vi "Read Background.vi"(8 "error in (no error)":errorcluster, 10 "Path":path, 11 "BigMAQ in":refnum<class "BigMAQ.lvclass">) -> (0 "error out":errorcluster, 3 "BigMAQ out":refnum<class "BigMAQ.lvclass">, 4 "Metadata":variant)   [LabVIEW 2019, in "BigMAQ.lvclass"]
uses:
  BigMAQ.lvclass
  BigMAQ.lvclass/BigMAQ.ctl
  <vilib>/vision/NI_Vision_Development_Module.lvlib
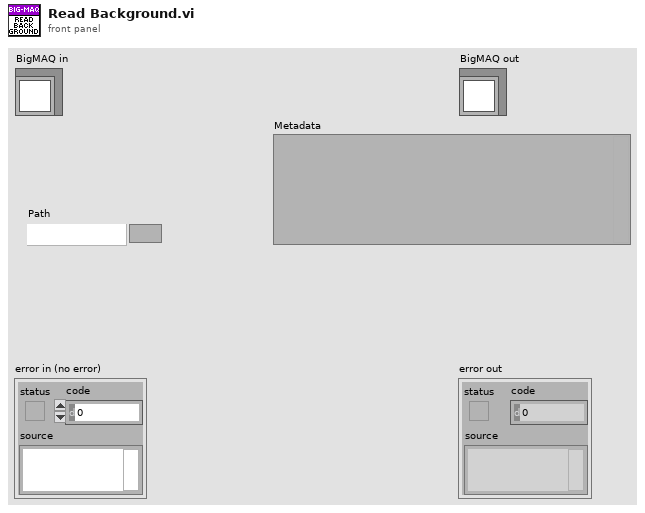
[diagram p1: front panel]
types:
  T1 = typedef "IMAQ Image.ctl" = refnum<image>
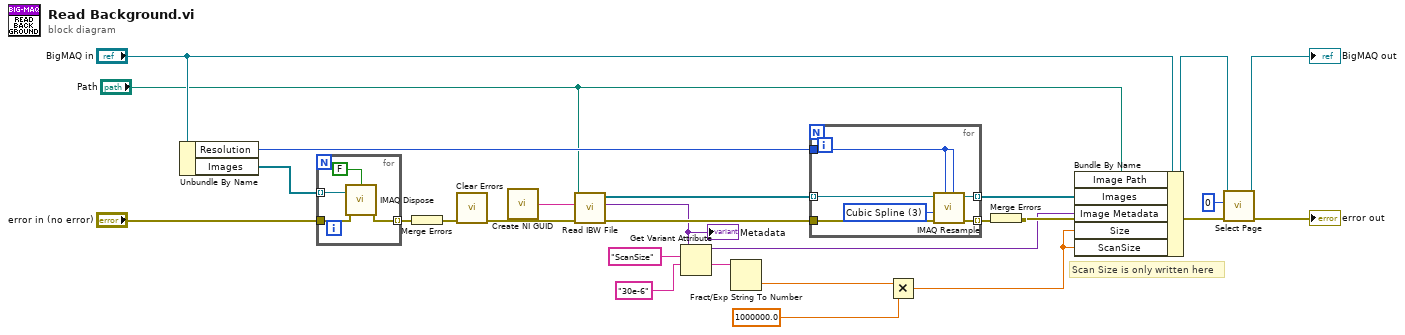
[diagram p0: block diagram]
diagram:
  # "Scan Size is only written here"
  n1 = Unbundle By Name("BigMAQ in") -> ("Resolution"=w20:i32, "Images"=w7:T1[])
  n2 = for {
    tunnel: w7 -> [w30] mode=indexing
    tunnel: [w29] -> w10 mode=indexing
    tunnel: "error in (no error)" -> [w28]
    n3 = call "IMAQ Dispose"("All Images? (No)"=FALSE, "Image"=w30, "error in (no error)"=w28) -> ("error out"=w29:errorcluster)  [unwired: 3 in]
  }
  n4 = Merge Errors(w10) -> (w8:errorcluster)
  n5 = call <vilib>:"Clear Errors.vi"("error in (no error)"=w8) -> ("error out"=w6:errorcluster)  [unwired: 5 in, 1 out]
  n6 = call "Create NI GUID.vi"() -> ("NI GUID"=w5:string)
  n7 = call "Read IBW File.vi"("error in (no error)"=w6, "Basename"=w5, "Path"="Path") -> ("error out"=w19:errorcluster, "Notes LUT"=w3:variant, "IMAQ"=w21:T1[])  [unwired: 6 in]
  "Metadata" <- w3
  n8 = Get Variant Attribute(Variant=w3, name="ScanSize", default value (empty Variant)="30e-6" ("name")) -> (duplicate Variant=w2:variant, value=w24:string)  [unwired: 1 in, 2 out]
  n9 = Fract/Exp String To Number(string=w24) -> (number=w22:dbl)  [unwired: 3 in, 1 out]
  n10 = for {
    tunnel: w21 -> [w35] mode=indexing
    tunnel: [w36] -> w17 mode=indexing
    tunnel: w20 -> [w33]
    tunnel: [w32] -> w18 mode=indexing
    tunnel: w19 -> [w31]
    w34 = u32 3 items=["Zero Order", "Bi-Linear", "Quadratic", "Cubic Spline"] ("Interpolation Type")
    n11 = call "IMAQ Resample"("X Resolution"=w33, "Y Resolution"=w33, "error in (no error)"=w31, "Interpolation Type"=w34, "Image Src"=w35) -> ("error out"=w32:errorcluster, "Image Dst Out"=w36:T1)  [unwired: 5 in]
  }
  n12 = Multiply(x=w22, y=1000000.0) -> (x*y=w1:dbl)
  n13 = Merge Errors(w18) -> (w16:errorcluster)
  n14 = Bundle By Name(cluster="BigMAQ in", "Image Path"="Path", "Images"=w17, "Image Metadata"=w2, "Size"=w1, "ScanSize"=w1) -> (w14:refnum<class "BigMAQ.lvclass">)
  n15 = call "Select Page.vi"("error in (no error)"=w16, "Page"=0, "BigMAQ in"=w14) -> ("error out"=→"error out":errorcluster, "BigMAQ out"=→"BigMAQ out":refnum<class "BigMAQ.lvclass">)  [unwired: 6 in, 1 out]
